vi "Read Digital In Status.vi"(8 "error in":errorcluster, 11 "MiniIO in":refnum<class "MiniIO.lvclass">) -> (0 "error out":errorcluster, 3 "MiniIO out":refnum<class "MiniIO.lvclass">)   [LabVIEW 2018, in "MiniIO.lvlib" / "MiniIO.lvclass"]
uses:
  MiniIO.lvclass
  MiniIO.lvclass/MiniIO.ctl
  <vilib>/NI/Modbus Library/API/Master/Modbus Master.lvclass
  PPLs/PLC/Parent/PLC.lvlibp/PLC.lvclass
  C:/AME Test Engineering/LabVIEW/PPLs/PLC/Parent/PLC.lvlibp/PLC.lvclass
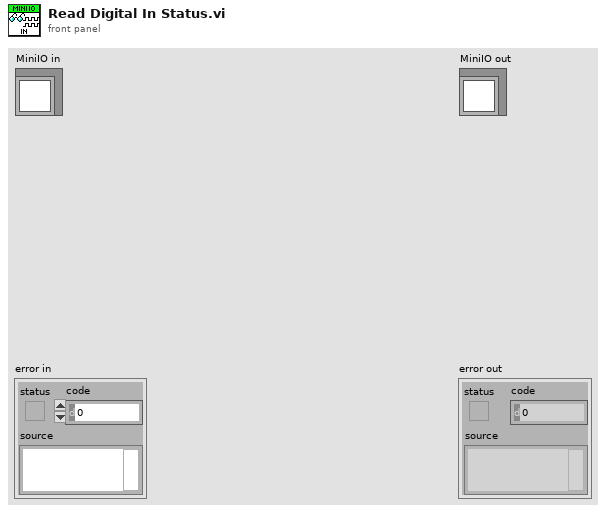
[diagram p1: front panel]
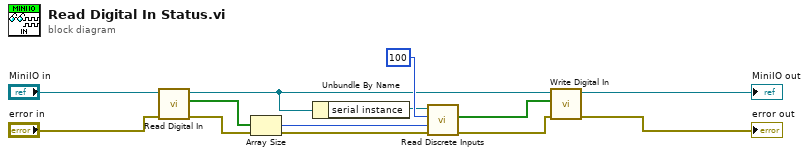
[diagram p0: block diagram]
diagram:
  n1 = call "Read Digital In.vi"("error in"="error in", "PLC in"="MiniIO in") -> ("error out"=w4:errorcluster, "Digital In"=w3:bool[], "PLC out"=w2:refnum<class "MiniIO.lvclass">)  [unwired: 7 in]
  n2 = Array Size(array=w3) -> (size(s)=w12:i32)
  n3 = Unbundle By Name(w2) -> ("serial instance"=w1:refnum<class "Modbus Master.lvclass">)
  n4 = call-dynamic "Read Discrete Inputs.vi"("error in"=w4, "number of inputs"=w12, "starting address"=u16 100, "Modbus master in"=w1) -> ("error out"=w8:errorcluster, "discrete inputs"=w7:bool[])  [unwired: 5 in, 1 out]
  n5 = call "Write Digital In.vi"("error in (no error)"=w8, "Digital In"=w7, "PLC in"=w2) -> ("error out"=→"error out":errorcluster, "PLC out"=→"MiniIO out":refnum<class "MiniIO.lvclass">)  [unwired: 7 in]
